vi "Temperature sensor.vi"(8 "error in":errorcluster) -> (0 "error out":errorcluster, 1 "Pass/Faile":bool, 2 "unsigned byte array":u8[](array[numeric]) format="%x", 3 "Tlcu Temp":dbl, 4 "Troom":string, 5 "Temp Address":string, 7 "communiction":bool)   [LabVIEW 2009]
uses:
  Digit IO PCI 6503/Digit IO control.ctl
  Global/Global 1.vi
  <vilib>/Instr/_visa.llb/VISA Configure Serial Port (Instr).vi
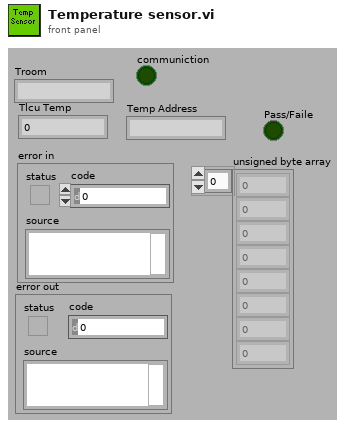
[diagram p1: front panel]
types:
  T1 = typedef "Digit IO control.ctl" = enum16{"Pull X1_4 Low", "Disconnect Pull X1_4 Low", "Down Cylinder", "Disconnect Down Cylinder", "Load X1_1_5", "Disconnect Load X1_1_5", "Measu X1_1_5", "Disconnect Measu X1_1_5", "Measu Z1_1_5", "Disconnect Measu Z1_1_5", "Power X1_1", "Disconnect Power X1_1", "RS232 Power", "Disconnect RS232 Power", "Card Cylinder", "Disconnect Card Cylinder", "Fail LED", "Disconnect Fail LED", "LCA Power", "Disconnect LCA Power", "BeyondCylinderDowndigit", "Disconnect BeyondCylinderDowendigit", "Frequency", "Disconnect Frequency", "Measu Current", "Disconnect Measu Current", "Measu current_1", "Disconnect Measu current_1", "Digit ALL", "Disconnect Digit ALL", "PASS LED", "Disconnect PASS LED", "Load Z1_1_3", "Disconnect Load Z1_1_3", "RS232 Connect", "Disconnect RS232 Connect", "Power Z1_7", "Disconnect Power Z1_7", "Pull Z_1_5  low", "Disconnect Pull Z_1_5  low", "Connect LCA_1", "Disconnect LCA_1", "short LCA", "Disconnect short LCA", "PT100", "Disconnect PT100", "NO connect", "Disconnect NO connect"}
  T2 = cluster{"VHEATFUSENOLOADMIN":string, "VHEATFUSELOADMAX":string, "VOVERRIDEDIODEMIN":string, "TDIFFMAX":string, "MEASFREQMAX":string, "MEASFREQMIN":string, "VOVER":string, "VMIDDLE":string, "VUNDER":string, "VNORESET":string, "VRESET":string, "WAITPING":string, "LRFID":string, "RFIDUID":string, "EXTEESIZE":string, "LCUTYPE":string, "LCUSUBTYPE":string, "TEVN":string, "BOOTVER":string, "APPVER":string, "ISLEEPMAX":string, "TSLEEP":string, "APPWAIT":string, "DBWAIT":string}
  T3 = cluster{"People":string, "product  number":string, "Test time":string, "VHeatFuse_noload":string, "VHeatFuse_load":string, "VoverrideDiode":string, "Test firmware upload via X1":string, "TemperAddress":string, "Troom":string, "TLCU":string, "Adjustment factor":string, "MeasuredFreq":string, "I2C communication":string, "Light-emitting diode on Z2":string, "Battery warning/inhibit":string, "Reset by IC10":string, "External EEPROM":string, "RFID card detection and reading RFID":string, "Production parameters in internal EEPROM":string, "Current consumption in sleep mode":string, "Application and database upload":string, "Test result":string, "Table head[22]":string, "Table head[23]":string}
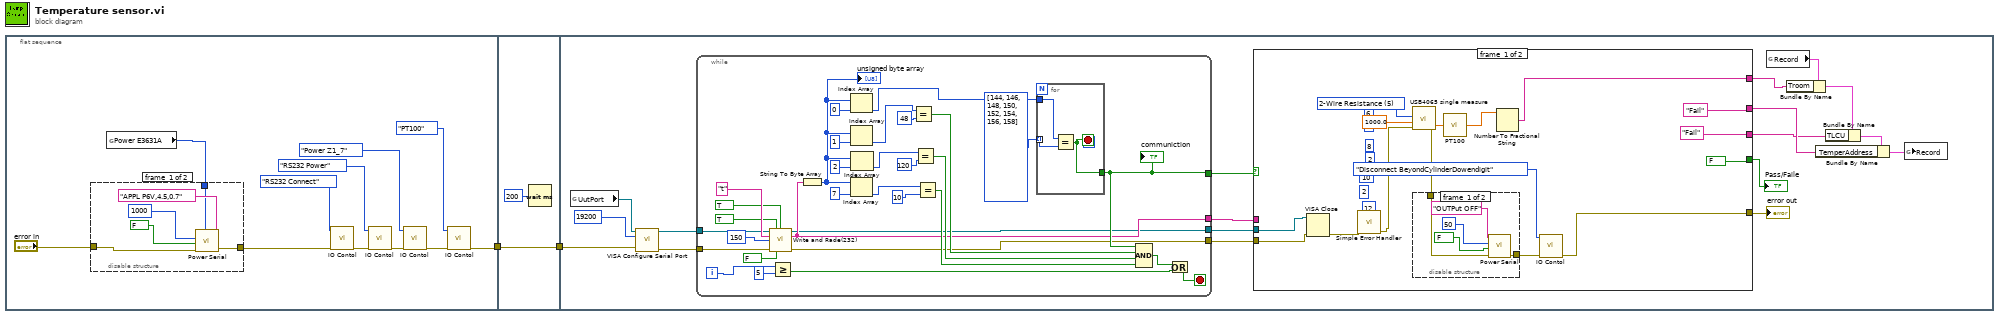
[diagram p0: block diagram]
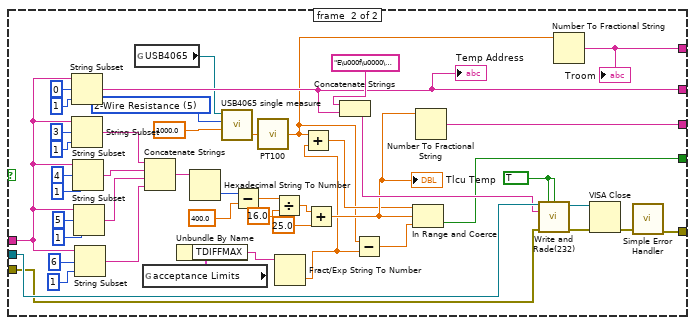
[diagram p4: hidden frame]
diagram:
  n1 = flat-sequence {
    tunnel: [w5] -> w1
    tunnel: w1 -> [w22]
    tunnel: [w22] -> w2
    tunnel: w2 -> [w23]
    frame #0 {
      n2 = global read "Global 1.vi" "Power E3631A"() -> (w12:i32)
      n3 = disable-structure shown="Enabled" {
        disable-tunnel: w12 -> [w16 _]
        disable-tunnel: [w15 w20] -> w10
        disable-tunnel: "error in" -> [w14 w20]
        frame #0 {
          n4 = call "Power Serial.vi"("VISA Resource Address"=w16, "error in (no error)"=w14, "Rd?"=FALSE, "Delay"=1000, "IN"="APPL P6V,4.5,0.7" ("In")) -> ("error out"=w15:errorcluster)  [unwired: 5 in, 1 out]
        }
        frame #1 {
        }
      }
      n5 = call "IO Contol.vi"("error in"=w10, "IO Operation"=Digit_IO_control."RS232 Connect" ("Enum")) -> ("error out"=w11:errorcluster)  [unwired: 9 out]
      n6 = call "IO Contol.vi"("error in"=w11, "IO Operation"=Digit_IO_control."RS232 Power" ("Enum")) -> ("error out"=w13:errorcluster)  [unwired: 9 out]
      n7 = call "IO Contol.vi"("error in"=w13, "IO Operation"=Digit_IO_control."Power Z1_7" ("Enum")) -> ("error out"=w6:errorcluster)  [unwired: 9 out]
      n8 = call "IO Contol.vi"("error in"=w6, "IO Operation"=Digit_IO_control."PT100") -> ("error out"=w5:errorcluster)  [unwired: 9 out]
    }
    frame #1 {
      n9 = Wait (ms)(milliseconds to wait=u32 200) -> ()  [unwired: 1 out]
    }
    frame #2 {
      (unwired) 12 ("offset (0)")
      (unwired) 10 ("offset (0)")
      (unwired) 8 ("offset (0)")
      (unwired) 6 ("offset (0)")
      (unwired) 2 ("length (rest)")
      (unwired) 2 ("length (rest)")
      (unwired) 2 ("length (rest)")
      (unwired) 2 ("length (rest)")
      n10 = global read "Global 1.vi" "UutPort"() -> (w24:refnum<visa-resource-name>)
      n11 = call-poly "VISA Configure Serial Port"("VISA resource name"=w24, "baud rate (9600)"=u32 19200, "error in (no error)"=w23) -> ("VISA resource name out"=w34:refnum<visa-resource-name>, "error out"=w35:errorcluster)  [unwired: 3 in, 8 out]
      n12 = while {
        tunnel: [w51] -> w39
        tunnel: [w64] -> w40
        tunnel: w35 -> [w47]
        tunnel: [w46] -> w38
        tunnel: w34 -> [w45]
        tunnel: [w44] -> w37
        i -> [w72]
        stop <- w65 stop-if-true
        n13 = call "Write and Rade(232).vi"("VISA resource name in"=w45, "write"=TRUE, "read"=TRUE, "string to write"="t", "ms delay"=u32 150 ("millisecond multiple"), "error in"=w47, "change baud rate(read)"=FALSE) -> ("VISA resource name out"=w44:refnum<visa-resource-name>, "read string"=w51:string, "error out"=w46:errorcluster)  [unwired: 1 in, 5 out]
        n14 = Greater Or Equal?(x=w72, y=5) -> (x >= y?=w67:bool)
        n15 = String To Byte Array(string=w51) -> (unsigned byte array=w59:u8[])
        "unsigned byte array" <- w59
        n16 = Index Array(array=w59, index=0) -> (element=w58:u8)
        n17 = Index Array(array=w59, index=1) -> (element=w57:u8)
        n18 = Index Array(array=w59, index=7) -> (element=w54:u8)
        n19 = Index Array(array=w59, index=2) -> (element=w55:u8)
        n20 = Equal?(x=w57, y=u8 48) -> (x = y?=w68:bool)
        n21 = Equal?(x=w55, y=u8 120) -> (x = y?=w69:bool)
        n22 = Equal?(x=w54, y=u8 10) -> (x = y?=w70:bool)
        n23 = for {
          tunnel: [w74] -> w64
          tunnel: w58 -> [w75]
          tunnel: u8[] [144, 146, 148, 150, 152, 154, 156, 158] -> [w73] mode=indexing
          stop <- w74 stop-if-true
          n24 = Equal?(x=w75, y=w73) -> (x = y?=w74:bool)
        }
        "communiction" <- w64
        n25 = Compound Arithmetic op=AND(w64, w68, w69, w70) -> (w66:bool)
        n26 = Or(x=w66, y=w67) -> (x .or. y?=w65:bool)
      }
      n27 = case shown="False" w40 {
        tunnel: w39 -> [_ w143]
        tunnel: [w90 w140] -> w33
        tunnel: w38 -> [w84 w141]
        tunnel: w37 -> [w85 w142]
        tunnel: [FALSE ("Rd?") w113] -> w32
        tunnel: ["Fail" w112] -> w30
        tunnel: ["Fail" w110] -> w29
        tunnel: [w76 w103] -> w25
        frame #0 {
          w82 = 5 items=["DC Volts"=1, "AC Volts"=2, "DC Current"=3, "AC Current"=4, "2-Wire Resistance"=5, "4-Wire Resistance"=101, "Frequency"=104, "Period"=105, "AC Volts DC Coupled"=1001, "Diode"=1002, "Waveform Voltage"=1003, "Waveform Current"=1004, "Capacitance"=1005, "Inductance"=1006, "Temperature"=108] ("Configuration:Function")
          n28 = VISA Close(VISA resource name=w85, error in (no error)=w84) -> (error out=w83:errorcluster)
          n29 = call <vilib>:"Simple Error Handler.vi"("error in (no error)"=w83) -> ("error out"=w79:errorcluster)  [unwired: 1 in, 7 out]
          n30 = call "USB4065 single measure.vi"("error in (no error)"=w79, "Configuration:Range"=1000.0, "Configuration:Function"=w82) -> ("error out"=w78:errorcluster, "Measurement"=w80:dbl)  [unwired: 1 in, 6 out]
          n31 = disable-structure shown="Enabled" {
            disable-tunnel: [w94 w97] -> w91
            disable-tunnel: w78 -> [w92 w97]
            frame #0 {
              n32 = call "Power Serial.vi"("error in (no error)"=w92, "Rd?"=FALSE, "Delay"=50, "IN"="OUTPut OFF" ("In")) -> ("error out"=w94:errorcluster)  [unwired: 6 in, 1 out]
            }
            frame #1 {
            }
          }
          n33 = call "PT100.vi"("R"=w80) -> ("T"=w77:dbl)
          n34 = Number To Fractional String(number=w77) -> (F-format string=w76:string)  [unwired: 3 out]
          n35 = call "IO Contol.vi"("error in"=w91, "IO Operation"=Digit_IO_control."Disconnect BeyondCylinderDowendigit" ("Enum")) -> ("error out"=w90:errorcluster)  [unwired: 9 out]
        }
        frame #1 {
          w109 = 5 items=["DC Volts"=1, "AC Volts"=2, "DC Current"=3, "AC Current"=4, "2-Wire Resistance"=5, "4-Wire Resistance"=101, "Frequency"=104, "Period"=105, "AC Volts DC Coupled"=1001, "Diode"=1002, "Waveform Voltage"=1003, "Waveform Current"=1004, "Capacitance"=1005, "Inductance"=1006, "Temperature"=108] ("Configuration:Function")
          w137 = TRUE ("write")
          n36 = String Subset(string=w143, offset (0)=0, length (rest)=1 ("length (rest)")) -> (substring=w112:string)
          "Temp Address" <- w112
          n37 = String Subset(string=w143, offset (0)=3, length (rest)=1 ("length (rest)")) -> (substring=w133:string)
          n38 = String Subset(string=w143, offset (0)=4, length (rest)=1 ("length (rest)")) -> (substring=w132:string)
          n39 = String Subset(string=w143, offset (0)=5, length (rest)=1 ("length (rest)")) -> (substring=w98:string)
          n40 = String Subset(string=w143, offset (0)=6, length (rest)=1 ("length (rest)")) -> (substring=w131:string)
          n41 = global read "Global 1.vi" "USB4065"() -> (w107:refnum<k15>)
          n42 = global read "Global 1.vi" "acceptance Limits"() -> (w101:T2)
          n43 = Concatenate Strings(w133, w132, w98, w131) -> (w116:string)
          n44 = Unbundle By Name(w101) -> ("TDIFFMAX"=w100:string)
          n45 = Hexadecimal String To Number(string=w116) -> (number=w130:u32)  [unwired: 3 out]
          n46 = call "USB4065 single measure.vi"("Configuration:Range"=1000.0, "Configuration:Function"=w109, "Instrument Descriptor"=w107) -> ("Measurement"=w106:dbl)  [unwired: 1 in, 7 out]
          n47 = Subtract(x=w130, y=400.0) -> (x-y=w128:dbl)
          n48 = call "PT100.vi"("R"=w106) -> ("T"=w102:dbl)
          n49 = Divide(x=w128, y=16.0) -> (x/y=w115:dbl)
          n50 = Fract/Exp String To Number(string=w100) -> (number=w99:dbl)  [unwired: 4 out]
          n51 = Add(x=w102, y=w99) -> (x+y=w105:dbl)
          n52 = Add(x=w115, y=25.0) -> (x+y=w111:dbl)
          "Tlcu Temp" <- w111
          n53 = Concatenate Strings("E\u000f\u0000\u0001" ("string"), w112) -> (w138:string)
          n54 = Subtract(x=w102, y=w99) -> (x-y=w104:dbl)
          n55 = In Range and Coerce(upper limit=w105, x=w111, lower limit=w104) -> (In Range?=w113:bool)  [unwired: 1 out]
          n56 = Number To Fractional String(number=w111) -> (F-format string=w110:string)  [unwired: 3 out]
          n57 = call "Write and Rade(232).vi"("VISA resource name in"=w142, "write"=w137, "read"=w137, "string to write"=w138, "error in"=w141) -> ("VISA resource name out"=w135:refnum<visa-resource-name>, "error out"=w136:errorcluster)  [unwired: 3 in, 6 out]
          n58 = Number To Fractional String(number=w102) -> (F-format string=w103:string)  [unwired: 3 out]
          "Troom" <- w103
          n59 = VISA Close(VISA resource name=w135, error in (no error)=w136) -> (error out=w134:errorcluster)
          n60 = call <vilib>:"Simple Error Handler.vi"("error in (no error)"=w134) -> ("error out"=w140:errorcluster)  [unwired: 1 in, 7 out]
        }
      }
      "error out" <- w33
      "Pass/Faile" <- w32
      n61 = global read "Global 1.vi" "Record"() -> (w27:T3)
      n62 = Bundle By Name(cluster=w27, "Troom"=w25) -> (w26:T3)
      n63 = Bundle By Name(cluster=w26, "TLCU"=w29) -> (w28:T3)
      n64 = Bundle By Name(cluster=w28, "TemperAddress"=w30) -> (w31:T3)
      n65 = global write "Global 1.vi" "Record"(w31) -> ()
    }
  }
